vi "Display 7 MC.vi"(0 "b0":bool, 2 "b1":bool, 3 "b3":bool, 4 "b2":bool) -> (1 "a":bool, 5 "b":bool, 6 "d":bool, 7 "e":bool, 8 "c":bool, 9 "f":bool, 10 "g":bool)   [LabVIEW 2012]
panel:
  out "L3":bool
  out "L 2":bool
  out "L1":bool
  out "L0":bool
  # "0"
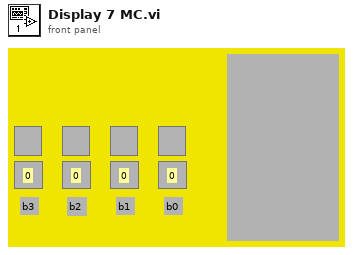
[diagram p1: front panel]
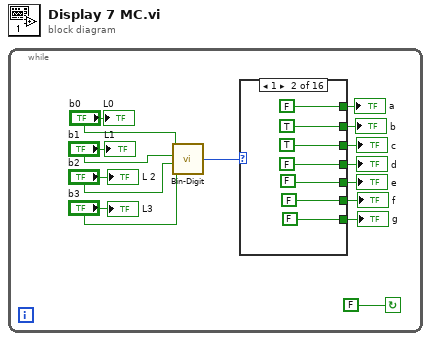
[diagram p0: block diagram]
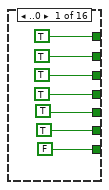
[diagram p2: hidden frame]
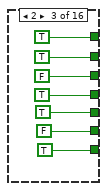
[diagram p3: hidden frame]
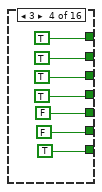
[diagram p4: hidden frame]
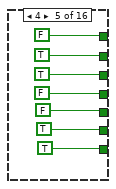
[diagram p5: hidden frame]
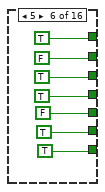
[diagram p6: hidden frame]
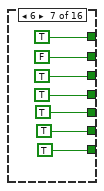
[diagram p7: hidden frame]
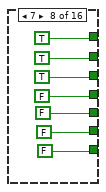
[diagram p8: hidden frame]
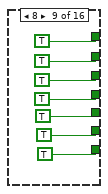
[diagram p9: hidden frame]
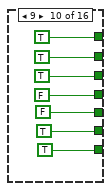
[diagram p10: hidden frame]
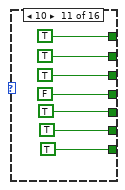
[diagram p11: hidden frame]
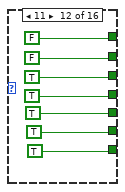
[diagram p12: hidden frame]
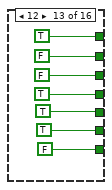
[diagram p13: hidden frame]
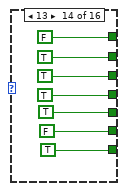
[diagram p14: hidden frame]
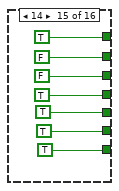
[diagram p15: hidden frame]
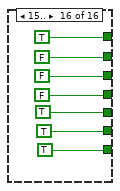
[diagram p16: hidden frame]
diagram:
  n1 = while {
    stop <- FALSE continue-if-true
    n2 = call "Bin-Digit.vi"("b3"="b3", "b2"="b2", "b1"="b1", "b0"="b0") -> ("Digit"=w6:i32)
    n3 = case shown="1" w6 {
      tunnel: [TRUE FALSE TRUE TRUE FALSE TRUE TRUE TRUE TRUE TRUE TRUE FALSE TRUE FALSE TRUE TRUE] -> w7
      tunnel: [TRUE TRUE TRUE TRUE TRUE FALSE FALSE TRUE TRUE TRUE TRUE FALSE FALSE TRUE FALSE FALSE] -> w8
      tunnel: [TRUE TRUE FALSE TRUE TRUE TRUE TRUE TRUE TRUE TRUE TRUE TRUE FALSE TRUE FALSE FALSE] -> w9
      tunnel: [TRUE FALSE TRUE TRUE FALSE TRUE TRUE FALSE TRUE FALSE FALSE TRUE TRUE TRUE TRUE FALSE] -> w10
      tunnel: [TRUE FALSE TRUE FALSE FALSE FALSE TRUE FALSE TRUE FALSE TRUE TRUE TRUE TRUE TRUE TRUE] -> w11
      tunnel: [TRUE FALSE FALSE FALSE TRUE TRUE TRUE FALSE TRUE TRUE TRUE TRUE TRUE FALSE TRUE TRUE] -> w12
      tunnel: [FALSE FALSE TRUE TRUE TRUE TRUE TRUE FALSE TRUE TRUE TRUE TRUE FALSE TRUE TRUE TRUE] -> w13
      frame ..0 {
      }
      frame 1 {
      }
      frame 2 {
      }
      frame 3 {
      }
      frame 4 {
      }
      frame 5 {
      }
      frame 6 {
      }
      frame 7 {
      }
      frame 8 {
      }
      frame 9 {
      }
      frame 10 {
      }
      frame 11 {
      }
      frame 12 {
      }
      frame 13 {
      }
      frame 14 {
      }
      frame 15.. {
      }
    }
    "e" <- w11
    "f" <- w12
    "c" <- w9
    "d" <- w10
    "g" <- w13
    "b" <- w8
    "a" <- w7
    "L0" <- "b0"
    "L1" <- "b1"
    "L 2" <- "b2"
    "L3" <- "b3"
  }
